vi "Test.vi"() -> ()   [LabVIEW 2014]
panel:
  out "appended array":cluster{"x":dbl, "y":dbl}[](array[cluster])
  out "array w/ subset deleted 2":cluster{"x":dbl, "y":dbl}[](array[cluster])
  out "array w/ subset deleted":cluster{"x":dbl, "y":dbl}[](array[cluster])
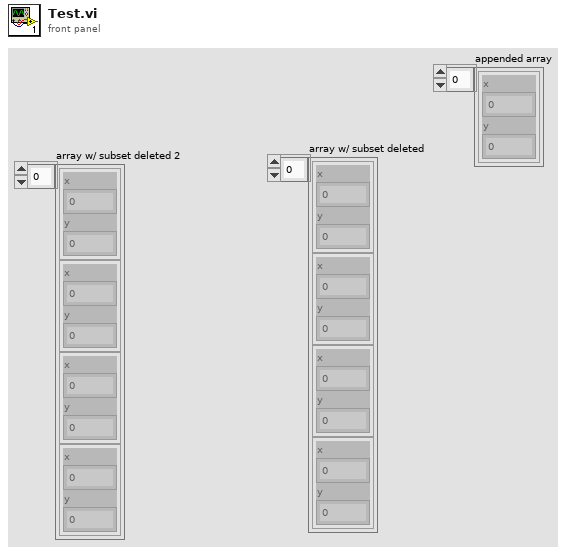
[diagram p1: front panel]
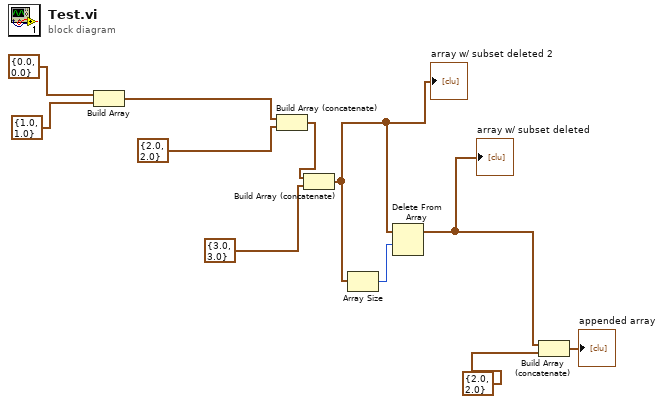
[diagram p0: block diagram]
diagram:
  n1 = Build Array(cluster{"x":dbl, "y":dbl} {"x"=0.0, "y"=0.0} ("Type - 2D Pose"), cluster{"x":dbl, "y":dbl} {"x"=1.0, "y"=1.0} ("Type - 2D Pose")) -> (w9:cluster{"x":dbl, "y":dbl}[])
  n2 = Build Array (concatenate)(w9, cluster{"x":dbl, "y":dbl} {"x"=2.0, "y"=2.0} ("Type - 2D Pose")) -> (w6:cluster{"x":dbl, "y":dbl}[])
  n3 = Build Array (concatenate)(w6, cluster{"x":dbl, "y":dbl} {"x"=3.0, "y"=3.0} ("Type - 2D Pose")) -> (w5:cluster{"x":dbl, "y":dbl}[])
  "array w/ subset deleted 2" <- w5
  n4 = Array Size(array=w5) -> (size(s)=w4:i32)
  n5 = Delete From Array(array=w5, length=w4) -> (array with subset deleted=w3:cluster{"x":dbl, "y":dbl}[])  [unwired: 1 in, 1 out]
  "array w/ subset deleted" <- w3
  n6 = Build Array (concatenate)(w3, cluster{"x":dbl, "y":dbl} {"x"=2.0, "y"=2.0} ("Type - 2D Pose")) -> (→"appended array":cluster{"x":dbl, "y":dbl}[])
